vi "Create  Input Pins Test Data.vi"(8 "错误输入":errorcluster, 11 "Pins Num":i32=1) -> (0 "错误输出":errorcluster, 3 "Data":bool[][](array[boolean]))   [LabVIEW 2012]
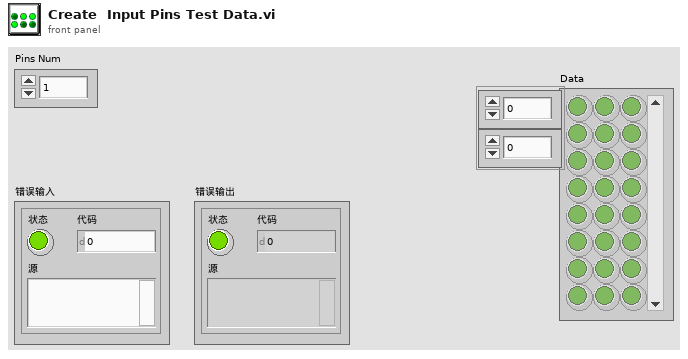
[diagram p1: front panel]
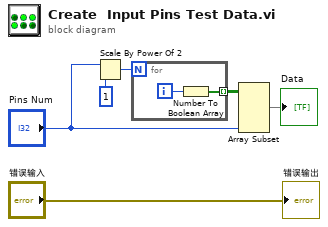
[diagram p0: block diagram]
diagram:
  n1 = Scale By Power Of 2(n="Pins Num", x=1) -> (x*2^n=w2:i32)
  n2 = for {
    N: w2 -> [_]
    tunnel: [w7] -> w4 mode=indexing
    i -> [w8]
    n3 = Number To Boolean Array(number=w8) -> (Boolean array=w7:bool[])
  }
  n4 = Array Subset(array=w4, length (col)="Pins Num") -> (→"Data":bool[][])  [unwired: 3 in]
  "错误输出" <- "错误输入"
